vi "DataIndicator_frontPanel.vi"() -> ()   [LabVIEW 2020]
panel:
  out "配列 2":string[][](array[string])
  in  "measurement condition output button":bool
  in  "Voltage":dbl(slide) scale=0.0..10.0
  in  "exposuretime":dbl(knob)=10.0 scale=0.0..10.0
  in  "unit":string="s"
  in  "comment":string
  in  "unit":string="um"
  in  "vslit":dbl=300.0
  in  "unit":string="um"
  in  "hslit":dbl
  in  "camera":string="Andor"
  in  "unit":string="Hz"
  in  "freq":string="0"
  in  "unit":string="mA"
  in  "compliance":dbl(slide) scale=-100.0..100.0
  in  "dcac":string="dc"
  in  "isBackconnector":bool
  in  "isFrontconnector":bool=TRUE
  in  "unit":string="mA"
  in  "current":dbl(slide) scale=-100.0..100.0
  in  "unit":string="v"
  in  "unit":string="Tesla"
  in  "magneticfield":dbl(slide) scale=-10.0..10.0
  in  "unit":string="K"
  in  "temperature":dbl(slide) scale=0.0..500.0
  in  "measureTime":string="1"
  out "date":string
  in  "fileType":string(combo)="uEL"
  in  "sampleMounting":string(combo)="422"
  in  "sampleName":string="QDL143(Omi)1"
  # "expos"
  # "temp"
  # "mag"
  # "curre"
  # "volt"
  # "NOT : 2byte character, symbol\nYES : english character"
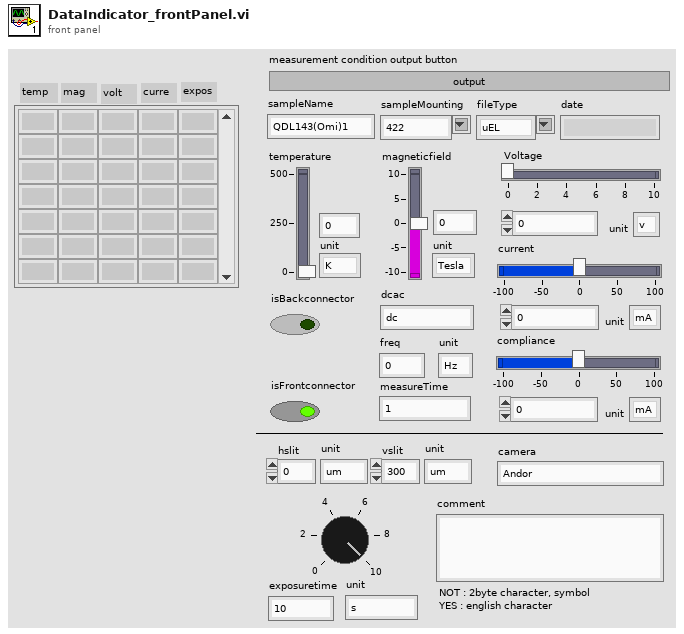
[diagram p1: front panel]
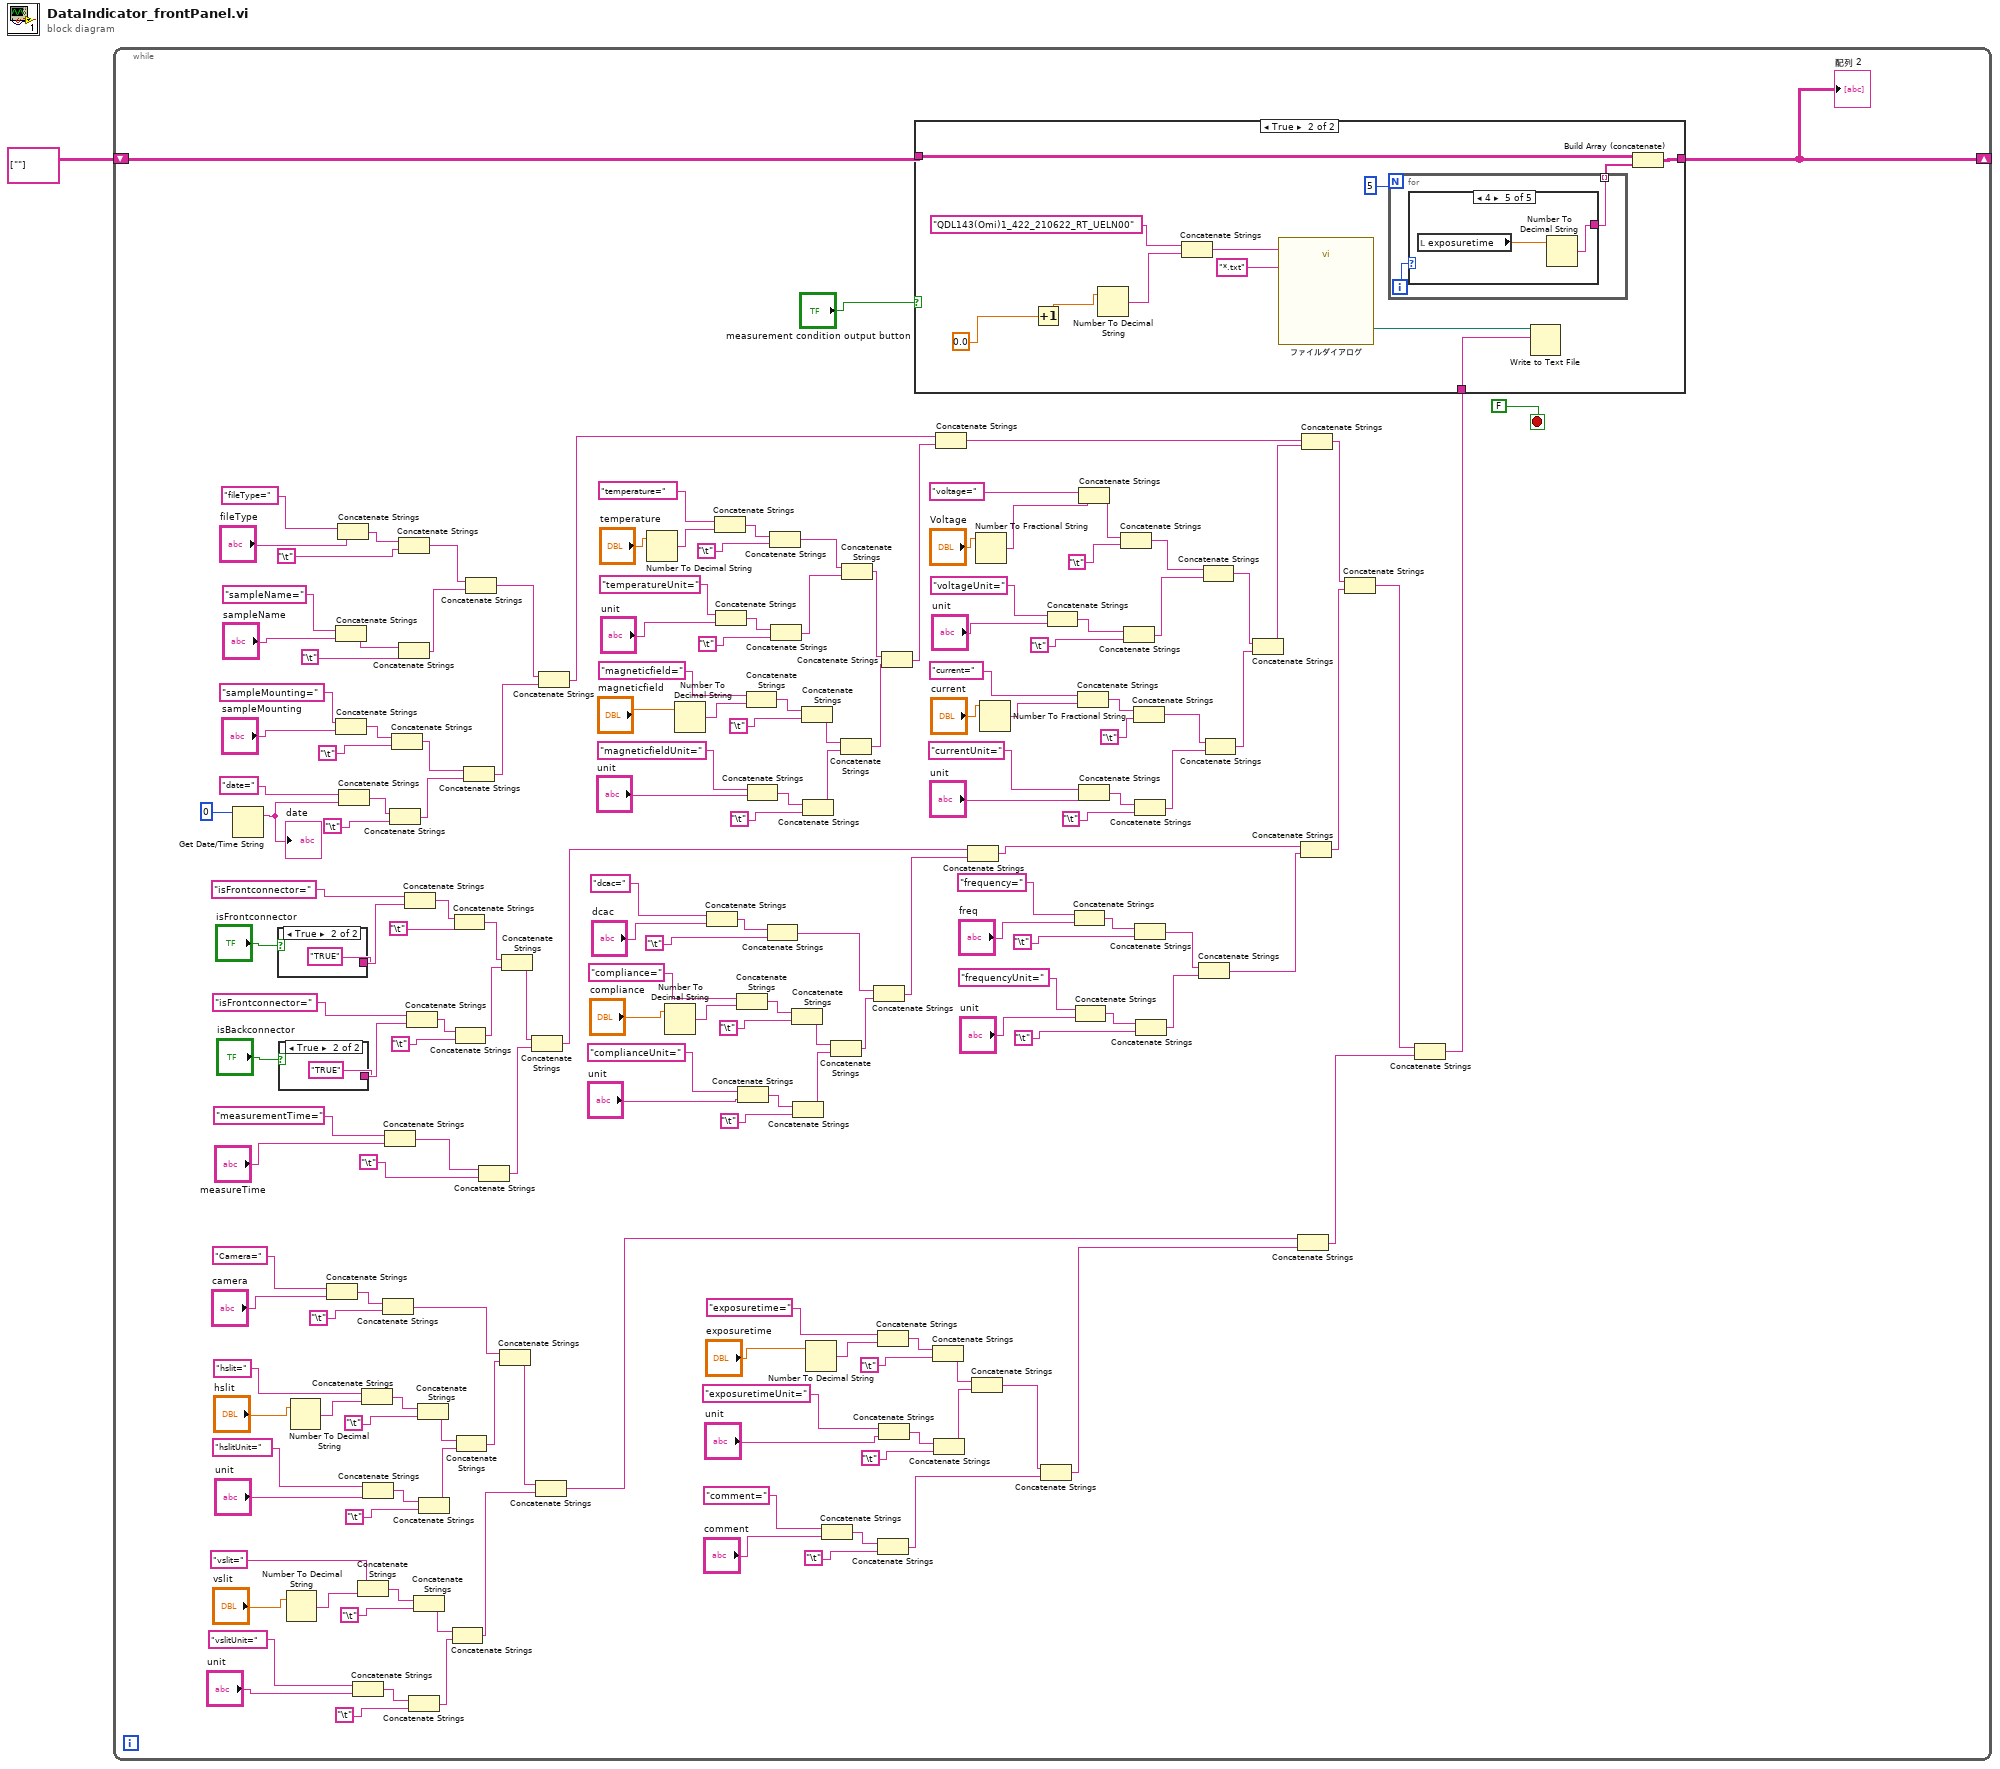
[diagram p0: block diagram]
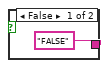
[diagram p2: hidden frame]
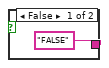
[diagram p3: hidden frame]
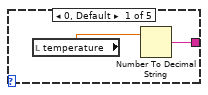
[diagram p5: hidden frame]
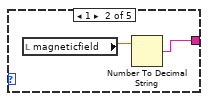
[diagram p6: hidden frame]
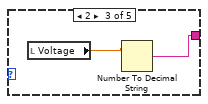
[diagram p7: hidden frame]
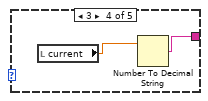
[diagram p8: hidden frame]
diagram:
  n1 = while {
    shift-right: [w5] -> _
    shift-left: string[][] [[""]] -> [w6]
    stop <- FALSE stop-if-true
    n2 = Get Date/Time String(date format (0)=0) -> (date string=w177:string)  [unwired: 2 in, 1 out]
    "date" <- w177
    n3 = case shown="TRUE" "isFrontconnector" {
      tunnel: ["FALSE" "TRUE"] -> w113
      frame False {
      }
      frame True {
      }
    }
    n4 = case shown="TRUE" "isBackconnector" {
      tunnel: ["FALSE" "TRUE"] -> w114
      frame False {
      }
      frame True {
      }
    }
    n5 = Number To Decimal String(number="vslit") -> (decimal integer string=w140:string)  [unwired: 1 in]
    n6 = Number To Decimal String(number="hslit") -> (decimal integer string=w133:string)  [unwired: 1 in]
    n7 = Concatenate Strings("Camera=", "camera") -> (w130:string)
    n8 = Concatenate Strings("sampleName=", "sampleName") -> (w73:string)
    n9 = Concatenate Strings("sampleMounting=", "sampleMounting") -> (w71:string)
    n10 = Concatenate Strings("fileType=", "fileType") -> (w78:string)
    n11 = Concatenate Strings("date=", w177) -> (w77:string)
    n12 = Concatenate Strings("vslitUnit=", "unit") -> (w180:string)
    n13 = Concatenate Strings("vslit=", w140) -> (w139:string)
    n14 = Concatenate Strings("hslit=", w133) -> (w132:string)
    n15 = Concatenate Strings("hslitUnit=", "unit") -> (w134:string)
    n16 = Concatenate Strings(w130, "\t") -> (w162:string)
    n17 = Concatenate Strings("measurementTime=", "measureTime") -> (w83:string)
    n18 = Concatenate Strings(w77, "\t") -> (w80:string)
    n19 = Concatenate Strings(w71, "\t") -> (w79:string)
    n20 = Concatenate Strings(w78, "\t") -> (w74:string)
    n21 = Concatenate Strings(w73, "\t") -> (w75:string)
    n22 = Concatenate Strings("isFrontconnector=", w113) -> (w111:string)
    n23 = Concatenate Strings("isFrontconnector=", w114) -> (w116:string)
    n24 = Concatenate Strings(w180, "\t") -> (w181:string)
    n25 = Concatenate Strings(w139, "\t") -> (w141:string)
    n26 = Concatenate Strings(w132, "\t") -> (w135:string)
    n27 = Concatenate Strings(w134, "\t") -> (w136:string)
    n28 = Concatenate Strings(w141, w181) -> (w165:string)
    n29 = Concatenate Strings(w111, "\t") -> (w150:string)
    n30 = Concatenate Strings(w116, "\t") -> (w151:string)
    n31 = Concatenate Strings(w135, w136) -> (w163:string)
    n32 = Concatenate Strings(w79, w80) -> (w81:string)
    n33 = Concatenate Strings(w74, w75) -> (w82:string)
    n34 = Concatenate Strings(w83, "\t") -> (w153:string)
    n35 = Concatenate Strings(w162, w163) -> (w164:string)
    n36 = Concatenate Strings(w150, w151) -> (w152:string)
    n37 = Concatenate Strings(w152, w153) -> (w156:string)
    n38 = Concatenate Strings(w164, w165) -> (w170:string)
    n39 = Concatenate Strings(w82, w81) -> (w9:string)
    n40 = Number To Decimal String(number="temperature") -> (decimal integer string=w7:string)  [unwired: 1 in]
    n41 = Number To Decimal String(number="compliance") -> (decimal integer string=w120:string)  [unwired: 1 in]
    n42 = Number To Decimal String(number="magneticfield") -> (decimal integer string=w91:string)  [unwired: 1 in]
    n43 = Concatenate Strings("dcac=", "dcac") -> (w117:string)
    n44 = Concatenate Strings("temperature=", w7) -> (w85:string)
    n45 = Concatenate Strings("temperatureUnit=", "unit") -> (w86:string)
    n46 = Concatenate Strings("compliance=", w120) -> (w119:string)
    n47 = Concatenate Strings("complianceUnit=", "unit") -> (w121:string)
    n48 = Concatenate Strings("magneticfield=", w91) -> (w90:string)
    n49 = Concatenate Strings("magneticfieldUnit=", "unit") -> (w92:string)
    n50 = Concatenate Strings(w117, "\t") -> (w154:string)
    n51 = Concatenate Strings(w85, "\t") -> (w88:string)
    n52 = Concatenate Strings(w86, "\t") -> (w89:string)
    n53 = Concatenate Strings(w119, "\t") -> (w122:string)
    n54 = Concatenate Strings(w121, "\t") -> (w123:string)
    n55 = Concatenate Strings(w90, "\t") -> (w93:string)
    n56 = Concatenate Strings(w92, "\t") -> (w94:string)
    n57 = Number To Decimal String(number="exposuretime") -> (decimal integer string=w144:string)  [unwired: 1 in]
    n58 = Concatenate Strings("comment=", "comment") -> (w166:string)
    n59 = Concatenate Strings(w122, w123) -> (w155:string)
    n60 = Concatenate Strings(w93, w94) -> (w107:string)
    n61 = Concatenate Strings(w88, w89) -> (w108:string)
    n62 = Concatenate Strings(w154, w155) -> (w157:string)
    n63 = Concatenate Strings("exposuretime=", w144) -> (w143:string)
    n64 = Concatenate Strings(w166, "\t") -> (w169:string)
    n65 = Concatenate Strings("exposuretimeUnit=", "unit") -> (w145:string)
    n66 = Concatenate Strings(w108, w107) -> (w10:string)
    n67 = Concatenate Strings(w143, "\t") -> (w146:string)
    n68 = Concatenate Strings(w145, "\t") -> (w147:string)
    n69 = Concatenate Strings(w9, w10) -> (w8:string)
    n70 = Concatenate Strings(w156, w157) -> (w161:string)
    n71 = Concatenate Strings(w146, w147) -> (w168:string)
    n72 = Number To Fractional String(number="Voltage") -> (F-format string=w3:string)  [unwired: 3 in]
    n73 = Number To Fractional String(number="current") -> (F-format string=w2:string)  [unwired: 3 in]
    n74 = Concatenate Strings(w168, w169) -> (w171:string)
    n75 = Concatenate Strings("voltageUnit=", "unit") -> (w98:string)
    n76 = Concatenate Strings("frequency=", "freq") -> (w126:string)
    n77 = Concatenate Strings("frequencyUnit=", "unit") -> (w128:string)
    n78 = Concatenate Strings("current=", w2) -> (w102:string)
    n79 = Concatenate Strings("voltage=", w3) -> (w97:string)
    n80 = Concatenate Strings("currentUnit=", "unit") -> (w103:string)
    n81 = Concatenate Strings(w97, "\t") -> (w99:string)
    n82 = Concatenate Strings(w98, "\t") -> (w100:string)
    n83 = Concatenate Strings(w102, "\t") -> (w104:string)
    n84 = Concatenate Strings(w103, "\t") -> (w105:string)
    n85 = Concatenate Strings(w126, "\t") -> (w158:string)
    n86 = Concatenate Strings(w128, "\t") -> (w159:string)
    n87 = Concatenate Strings(w158, w159) -> (w160:string)
    n88 = Concatenate Strings(w99, w100) -> (w109:string)
    n89 = Concatenate Strings(w104, w105) -> (w110:string)
    n90 = Concatenate Strings(w109, w110) -> (w12:string)
    n91 = Concatenate Strings(w170, w171) -> (w173:string)
    n92 = Concatenate Strings(w161, w160) -> (w172:string)
    n93 = Concatenate Strings(w8, w12) -> (w11:string)
    n94 = Concatenate Strings(w11, w172) -> (w174:string)
    n95 = Concatenate Strings(w174, w173) -> (w4:string)
    n96 = case shown="TRUE" "measurement condition output button" {
      tunnel: w4 -> [_ w191]
      tunnel: [w188 w193] -> w5
      tunnel: w6 -> [w188 w192]
      frame False {
      }
      frame True {
        n97 = Increment(x=0.0) -> (x+1=w196:dbl)
        n98 = Number To Decimal String(number=w196) -> (decimal integer string=w197:string)  [unwired: 1 in]
        n99 = Concatenate Strings("QDL143(Omi)1_422_210622_RT_UELN00", w197) -> (w198:string)
        n100 = call "ファイルダイアログ"("default name"=w198, "pattern (all files)"="*.txt" ("文字列 2")) -> ("selected path"=w199:path)  [unwired: 10 in, 3 out]
        n101 = for {
          N: 5 -> [_]
          tunnel: [w201] -> w190 mode=indexing
          i -> [w202]
          n102 = case shown="4" w202 {
            tunnel: [w203 w205 w207 w209 w211] -> w201
            frame 0, Default {
              n103 = local read "temperature"() -> (w204:dbl)
              n104 = Number To Decimal String(number=w204) -> (decimal integer string=w203:string)  [unwired: 1 in]
            }
            frame 1 {
              n105 = local read "magneticfield"() -> (w206:dbl)
              n106 = Number To Decimal String(number=w206) -> (decimal integer string=w205:string)  [unwired: 1 in]
            }
            frame 2 {
              n107 = local read "Voltage"() -> (w208:dbl)
              n108 = Number To Decimal String(number=w208) -> (decimal integer string=w207:string)  [unwired: 1 in]
            }
            frame 3 {
              n109 = local read "current"() -> (w210:dbl)
              n110 = Number To Decimal String(number=w210) -> (decimal integer string=w209:string)  [unwired: 1 in]
            }
            frame 4 {
              n111 = local read "exposuretime"() -> (w212:dbl)
              n112 = Number To Decimal String(number=w212) -> (decimal integer string=w211:string)  [unwired: 1 in]
            }
          }
        }
        n113 = Write to Text File(file (use dialog)=w199, text=w191) -> ()  [unwired: 2 in, 3 out]
        n114 = Build Array (concatenate)(w192, w190) -> (w193:string[][])
      }
    }
    "配列 2" <- w5
  }
